vi "final_control_mk5_022625.vi"() -> ()   [LabVIEW 2023]
doc: "Simplified example program for initializing the COM port, determining the data frame of up to 26 Alicats, acquiring the data of the same number of Alicats, displaying the data of the one with the selected unit ID, and writing a setpoint to the same selected unit ID.\n\nThis is a slightly more feature rich version of the Alicat Simplified Driver Example, and contains an example of a method for interfacing with up to 26 Alicats on a single COM port by means of for loops with shift registers to handle sequential commands to each included Alicat. This also contains a method to write a setpoint to the same selected unit.\n\nIf coding for multiple Alicats on a single COM port without the use of for loops with shift registers, ensure that each Alicat command is executed sequentially. Alicat's RS-232/485 does not work if multiple devices are responding simultaneously."
uses:
  <vilib>/Platform/TimedLoop/XDataNode/timing_clust.ctl
  <vilib>/Platform/TimedLoop/XDataNode/nitl_modes.ctl
  <vilib>/Platform/TimedLoop/XDataNode/wakeup.ctl
  <vilib>/DAQmx/write.llb/DAQmx Write (Analog 1D DBL NChan 1Samp).vi
  <vilib>/DAQmx/read.llb/DAQmx Read (Analog 1D DBL 1Chan NSamp).vi
  <extravilib>/ChannelInstances/Tag-bool/Read With Abort.vi
  <extravilib>/ChannelInstances/Tag-bool/Write With Abort.vi
  <vilib>/Utility/file.llb/Write Delimited Spreadsheet (string).vi
  <extravilib>/ChannelInstances/Tag-bool/Instantiate.vi
  <vilib>/Utility/file.llb/Read Delimited Spreadsheet (DBL).vi
  <extravilib>/ChannelInstances/Tag-bool/EndpointRead.vi
  <vilib>/DAQmx/miscellaneous.llb/DAQmx Fill In Error Info.vi
  <extravilib>/ChannelInstances/Tag-bool/Endpoint.vi
  <vilib>/platform/TimedLoop/XDataNode/XDataNode.xnode
  <vilib>/Platform/TimedLoop/XDataNode/XDNodeRunTimeDep.lvlib
  <extravilib>/ChannelInstances/Tag-bool.lvlib
panel:
  in  "Tab Control":enum32{"Page 1", "Page 2"}(tab)
  in  "COM Port Settings":T1={"Baud Rate"=enum."19200", "VISA Sesssion In"="COM1"}
  out "Range Exceeded":bool
  out "Error Present":bool
  out "Error Text":string
  out "Elapsed Time [ms]\n(all units)":dbl caption="Elapsed Time (s)"
  in  "Minimum time between \nreadings [ms] (all units)":u32
  in  "Device ID's \nto Include:":T2={"A"=TRUE, "B"=TRUE, "C"=TRUE, "D"=TRUE, "E"=TRUE, "F"=TRUE, "G"=FALSE, "H"=FALSE, "I"=FALSE, "J"=FALSE, "K"=FALSE, "L"=FALSE, "M"=FALSE, "N"=FALSE, "O"=FALSE, "P"=FALSE, "Q"=FALSE, "R"=FALSE, "S"=FALSE, "T"=FALSE, "U"=FALSE, "V"=FALSE, "W"=FALSE, "X"=FALSE, "Y"=FALSE, "Z"=FALSE}
  out "Active Device":u16(ring) items=["A", "B", "C", "D", "E", "F"]
  out "Meas. Data (for active device)":T3
  in  "Write File":path=path "C:/Users/gtmiller/Downloads/Alicat LabVIEW 2014_2v1/Test.csv"
  in  "Hold Time [min]":dbl=17.0 min=17.0
  out "Global Start Time":i64
  out "N":i32
  out "Iteration Duration":i64
  in  "Read File":path
  in  "End Program":bool
  out "len_SP":i32
  out "Setpoints":dbl[][](array[numeric])=[[4.2, 3.3], [69.0, 4.2]]
  out "Z":dbl[](array[numeric])
  out "ASP":dbl
  out "BSP":dbl
  out "CSP":dbl
  out "DSP":dbl
  out "ESP":dbl
  out "FSP":dbl
  out "N_i_read":dbl
  out "N_read":i32
  out "read count":dbl=2.0
  out "T_SCh":string[](array[string])
  out "Iter_#":string
  out "V_D":string
  out "V_H":string
  out "Iter_Duration":string
  # "Totalizer Timer"
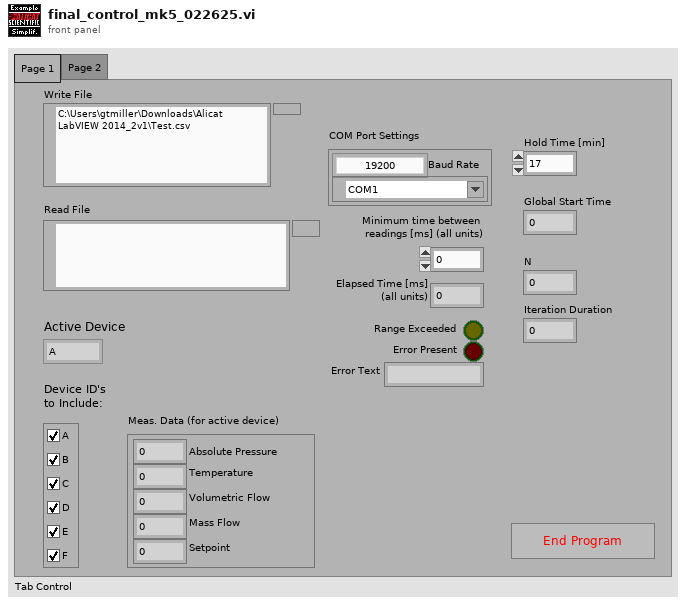
[diagram p1: front panel]
types:
  T1 = cluster{"Baud Rate":enum8{"2400", "9600", "19200", "38400", "57600", "115200", "Unknown"}, "VISA Sesssion In":refnum<visa-resource-name>}
  T2 = cluster{"A":bool, "B":bool, "C":bool, "D":bool, "E":bool, "F":bool, "G":bool, "H":bool, "I":bool, "J":bool, "K":bool, "L":bool, "M":bool, "N":bool, "O":bool, "P":bool, "Q":bool, "R":bool, "S":bool, "T":bool, "U":bool, "V":bool, "W":bool, "X":bool, "Y":bool, "Z":bool}
  T3 = cluster{"Absolute Pressure":dbl, "Gauge/Diff. Pressure":dbl, "Barometric Pressure":dbl, "Temperature":dbl, "Volumetric Flow":dbl, "Mass Flow":dbl, "Setpoint":dbl, "Valve Drive":dbl, "Totalizer":dbl, "[hr]":dbl, "[min]":dbl, "[sec]":dbl, "Totalizer Average Flow":dbl, "Totalizer Peak Flow":dbl, "Gas selected":string}
  T4 = cluster{"Unit ID":string, "Baud Rate":enum8{"2400", "9600", "19200", "38400", "57600", "115200", "Unknown"}, "VISA Sesssion In":refnum<visa-resource-name>}
  T5 = typedef "XDNodeRunTimeDep.lvlib/timing_clust.ctl" = cluster{"Expected End [f-1]":u64, "Actual End [f-1]":u64, "Finished Late? [f-1]":bool, "Expected End [i-1]":u64, "Actual End [i-1]":u64, "Finished Late? [i-1]":bool, "Expected Start [i]":u64, "Actual Start [i]":u64, "Expected Start [f]":u64, "Actual Start [f]":u64, "Source Name":string, "Structure Name":string, "Period":i64, "Deadline":i64, "Offset":i64, "Start":i64, "Priority":i32, "Timeout":i32, "Mode":T6, "Wakeup Reason":T7, "Error":errorcluster, "Source Type":string, "Secondary Source Type":string, "Global End Time":u64, "Global Start Time":u64, "Frame Duration":u64, "Iteration Duration":u64, "Assigned CPU":i32, "I/O Scan Engine Mode":u32}
  T6 = typedef "XDNodeRunTimeDep.lvlib/nitl_modes.ctl" = enum32{"No Change", "Process missed periods, maintain original phase", "Discard missed periods, maintain original phase", "Process missed periods, ignore original phase", "Discard missed periods, ignore original phase"}
  T7 = typedef "XDNodeRunTimeDep.lvlib/wakeup.ctl" = enum32{"Normal", "Aborted", "Asynchronous wakeup", "Timing source error", "Timed loop error", "Timeout"}
  T8 = typedef "Tag-bool.lvlib/))Channel.ctl" = refnum<queue>
  T9 = enum8{"2400", "9600", "19200", "38400", "57600", "115200", "Unknown"}
  T10 = cluster{"Absolute Pressure":bool, "Gauge/Diff. Pressure":bool, "Barometric Pressure":bool, "Temperature":bool, "Volumetric":bool, "Mass":bool, "Setpoint":bool, "Valve Drive":bool, "Totalizer":bool, "Totalizer Timer":bool, "Totalizer Average Flow":bool, "Totalizer Peak Flow":bool, "Gas Selected":bool, "Tot. Timer Format":u16}
  T11 = cluster{"Controller Full Scale":dbl, "Controller Select":u16, "Control Range":enum16{"Normal", "Inverted", "Bidirectional", "Unknown"}}
  T12 = cluster{"Controller Full Scale":dbl, "Controller Select":u16, "Control Range":enum16{"Normal", "Inverted", "Bidirectional", "Unknown"}}[]
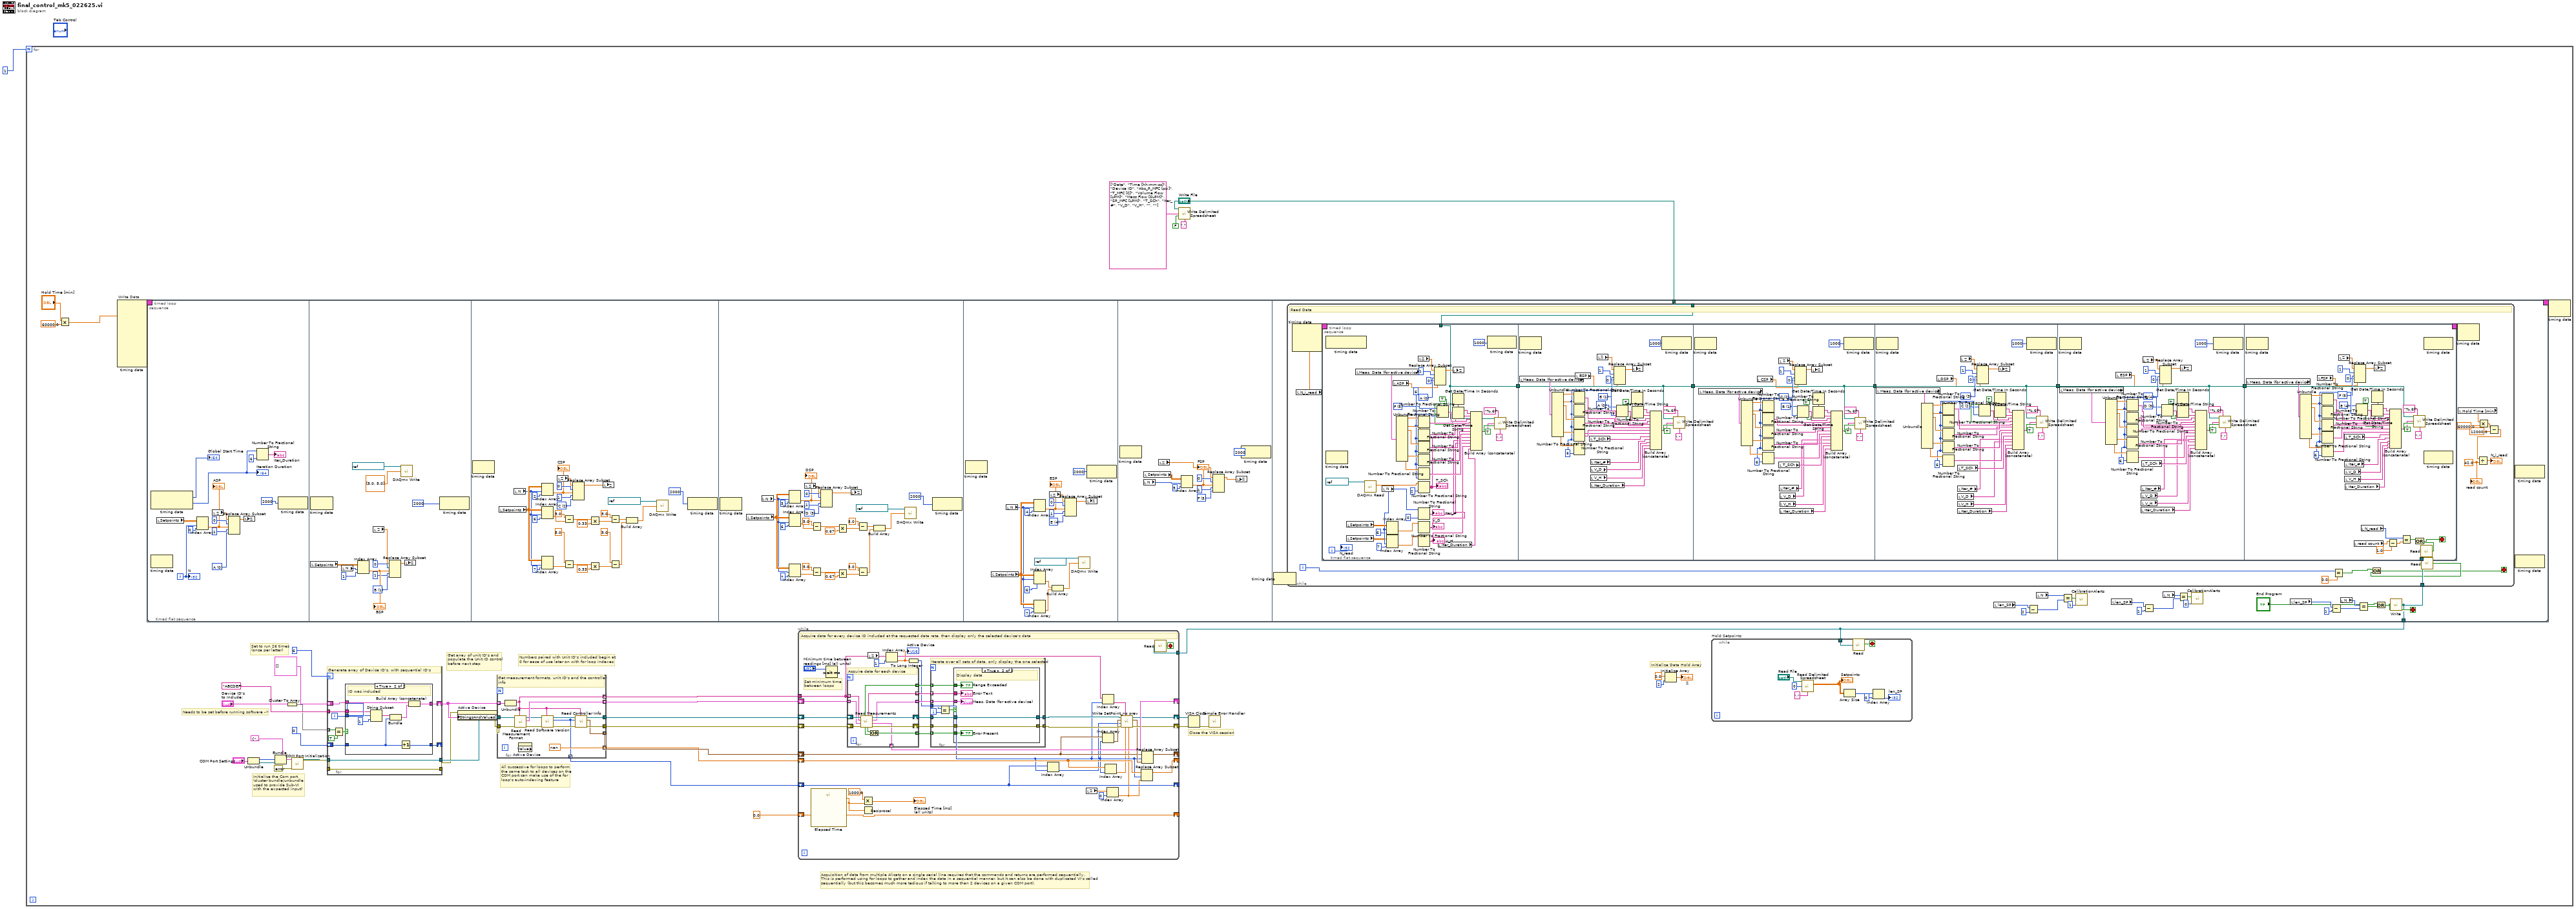
[diagram p0: block diagram]
diagram:
  n1 = for {
    N: 1 -> [_]
    # "Initialize Data Hold Array"
    # "All successive for loops to perform\nthe same task to all devices on the\nCOM port can make use of the for\nloop's auto-indexing feature"
    # "Set to run 26 times\n(once per letter)"
    # "Acquisition of data from multiple Alicats on a single serial line requires that the commands and returns are performed sequentially.\nThis is performed using for loops to gather and index the data in a sequential manner, but it can also be done with duplicated VI's called\nsequentially (but this becomes much more tedious if talking to more than 2 devices on a given COM port)."
    # "Numbers paired with Unit ID's included begin at\n0 for ease of use later on with for loop indexes"
    # "Get array of unit ID's and populate the Unit ID control before next step"
    # "Needs to be set before running software ->"
    # "Close the VISA session"
    # "Initialize the Com port\n(cluster bundle/unbundle\nused to provide Sub-VI \nwith the expected input)"
    n2 = Multiply(x="Hold Time [min]", y=60000.0) -> (x*y=w2:dbl)
    n3 = node-c288(w2) -> (w43:T5)  [unwired: 9 in]
    n4 = timed-loop "Write Data" {
      timing: w43 -> [_]
      timing-out: [_] -> w42
      tunnel: [w54] -> w9
      tunnel: "Write File" -> [w53]
      i -> [w68]
      stop <- w208 stop-if-true
      n5 = timed-sequence {
        timing: _ -> [_]
        timing-out: _ -> [_]
        tunnel: [w56] -> w54
        tunnel: w53 -> [w55]
        n6 = timed-flat-sequence {
          tunnel: [w203] -> w56
          tunnel: w55 -> [w204]
          frame #0 {
            w61 = u16 0 items=["A", "B", "C", "D", "E", "F"]
            n7 = node-c288() -> (→"Global Start Time":i64, w60:i64)  [unwired: 1 in]
            "Iteration Duration" <- w60
            n8 = local read "Setpoints"() -> (w70:dbl[][])
            n9 = Index Array(array=w70, index (row)=w68, index (col)=0 ("index (row)")) -> (element=w66:dbl)
            "ASP" <- w66
            n10 = local read "Z"() -> (w64:dbl[])
            n11 = Replace Array Subset(array=w64, new element #1=w66, index #1=0 ("index"), new element #2=w61, index #2=1 ("index")) -> (w65:dbl[])
            n12 = local write "Z"(w65) -> ()
            n13 = Number To Fractional String(number=w60, precision (6)=i16 6) -> (F-format string=→"Iter_Duration":string)  [unwired: 2 in]
            n14 = node-c288(i64 2000 ("Start")) -> ()  [unwired: 1 out]
            "N" <- w68
          }
          frame #1 {
            w79 = u16 1 items=["A", "B", "C", "D", "E", "F"]
            n15 = node-c288() -> ()  [unwired: 1 in, 1 out]
            n16 = local read "Setpoints"() -> (w87:dbl[][])
            n17 = local read "N"() -> (w80:i32)
            n18 = Index Array(array=w87, index (row)=w80, index (col)=1 ("index (row)")) -> (element=w84:dbl)
            "BSP" <- w84
            n19 = local read "Z"() -> (w82:dbl[])
            n20 = Replace Array Subset(array=w82, new element #1=w84, index #1=0 ("index"), new element #2=w79, index #2=1 ("index")) -> (w83:dbl[])
            n21 = call-poly <vilib>:"DAQmx Write.vi"("task/channels in"=refnum<k21> "Valve_cont", "data"=dbl[] [5.0, 5.0]) -> ()  [unwired: 11 in, 3 out]
            n22 = local write "Z"(w83) -> ()
            n23 = node-c288(i64 2000 ("Start")) -> ()  [unwired: 1 out]
          }
          frame #2 {
            w113 = u16 2 items=["A", "B", "C", "D", "E", "F"]
            n24 = node-c288() -> ()  [unwired: 1 in, 1 out]
            n25 = local read "Setpoints"() -> (w96:dbl[][])
            n26 = local read "N"() -> (w95:i32)
            n27 = Index Array(array=w96, index (row)=w95, index (col)=2 ("index (row)")) -> (element=w117:dbl)
            "CSP" <- w117
            n28 = Index Array(array=w96, index (row)=w95, index (col)=6 ("disabled index (col)")) -> (element=w94:dbl)
            n29 = Index Array(array=w96, index (row)=w95, index (col)=7 ("disabled index (col)")) -> (element=w93:dbl)
            n30 = local read "Z"() -> (w115:dbl[])
            n31 = Subtract(x=5.0, y=w94) -> (x-y=w110:dbl)
            n32 = Subtract(x=5.0, y=w93) -> (x-y=w105:dbl)
            n33 = Replace Array Subset(array=w115, new element #1=w117, index #1=0 ("index"), new element #2=w113, index #2=1 ("index")) -> (w116:dbl[])
            n34 = Multiply(x=w110, y=0.33) -> (x*y=w108:dbl)
            n35 = Multiply(x=w105, y=0.33) -> (x*y=w103:dbl)
            n36 = local write "Z"(w116) -> ()
            n37 = Subtract(x=5.0, y=w108) -> (x-y=w98:dbl)
            n38 = Subtract(x=5.0, y=w103) -> (x-y=w99:dbl)
            n39 = Build Array(w98, w99) -> (w97:dbl[])
            n40 = call-poly <vilib>:"DAQmx Write.vi"("task/channels in"=refnum<k21> "Valve_cont", "data"=w97) -> ()  [unwired: 11 in, 3 out]
            n41 = node-c288(i64 2000 ("Start")) -> ()  [unwired: 1 out]
          }
          frame #3 {
            w145 = u16 3 items=["A", "B", "C", "D", "E", "F"]
            n42 = node-c288() -> ()  [unwired: 1 in, 1 out]
            n43 = local read "Setpoints"() -> (w128:dbl[][])
            n44 = local read "N"() -> (w127:i32)
            n45 = Index Array(array=w128, index (row)=w127, index (col)=3 ("index (row)")) -> (element=w149:dbl)
            "DSP" <- w149
            n46 = Index Array(array=w128, index (row)=w127, index (col)=6 ("disabled index (col)")) -> (element=w126:dbl)
            n47 = Index Array(array=w128, index (row)=w127, index (col)=7 ("disabled index (col)")) -> (element=w125:dbl)
            n48 = local read "Z"() -> (w147:dbl[])
            n49 = Subtract(x=5.0, y=w126) -> (x-y=w142:dbl)
            n50 = Subtract(x=5.0, y=w125) -> (x-y=w137:dbl)
            n51 = Replace Array Subset(array=w147, new element #1=w149, index #1=0 ("index"), new element #2=w145, index #2=1 ("index")) -> (w148:dbl[])
            n52 = Multiply(x=w142, y=0.67) -> (x*y=w140:dbl)
            n53 = Multiply(x=w137, y=0.67) -> (x*y=w135:dbl)
            n54 = local write "Z"(w148) -> ()
            n55 = Subtract(x=5.0, y=w140) -> (x-y=w130:dbl)
            n56 = Subtract(x=5.0, y=w135) -> (x-y=w131:dbl)
            n57 = Build Array(w130, w131) -> (w129:dbl[])
            n58 = call-poly <vilib>:"DAQmx Write.vi"("task/channels in"=refnum<k21> "Valve_cont", "data"=w129) -> ()  [unwired: 11 in, 3 out]
            n59 = node-c288(i64 2000 ("Start")) -> ()  [unwired: 1 out]
          }
          frame #4 {
            w166 = u16 4 items=["A", "B", "C", "D", "E", "F"]
            n60 = node-c288() -> ()  [unwired: 1 in, 1 out]
            n61 = local read "Setpoints"() -> (w160:dbl[][])
            n62 = local read "N"() -> (w159:i32)
            n63 = Index Array(array=w160, index (row)=w159, index (col)=4 ("index (row)")) -> (element=w170:dbl)
            "ESP" <- w170
            n64 = Index Array(array=w160, index (row)=w159, index (col)=6 ("disabled index (col)")) -> (element=w162:dbl)
            n65 = Index Array(array=w160, index (row)=w159, index (col)=7 ("disabled index (col)")) -> (element=w161:dbl)
            n66 = local read "Z"() -> (w168:dbl[])
            n67 = Build Array(w162, w161) -> (w158:dbl[])
            n68 = Replace Array Subset(array=w168, new element #1=w170, index #1=0 ("index"), new element #2=w166, index #2=1 ("index")) -> (w169:dbl[])
            n69 = call-poly <vilib>:"DAQmx Write.vi"("task/channels in"=refnum<k21> "Valve_cont", "data"=w158) -> ()  [unwired: 11 in, 3 out]
            n70 = local write "Z"(w169) -> ()
            n71 = node-c288(i64 2000 ("Start")) -> ()  [unwired: 1 out]
          }
          frame #5 {
            w180 = u16 5 items=["A", "B", "C", "D", "E", "F"]
            n72 = node-c288() -> ()  [unwired: 1 in, 1 out]
            n73 = local read "N"() -> (w178:i32)
            n74 = local read "Setpoints"() -> (w183:dbl[][])
            n75 = local read "Z"() -> (w182:dbl[])
            n76 = Index Array(array=w183, index (row)=w178, index (col)=5 ("index (row)")) -> (element=w179:dbl)
            "FSP" <- w179
            n77 = Replace Array Subset(array=w182, new element #1=w179, index #1=0 ("index"), new element #2=w180, index #2=1 ("index")) -> (w181:dbl[])
            n78 = local write "Z"(w181) -> ()
            n79 = node-c288(i64 2000 ("Start")) -> ()  [unwired: 1 out]
          }
          frame #6 {
            n80 = node-c288() -> ()  [unwired: 1 in, 1 out]
            n81 = local read "len_SP"() -> (w192:i32)
            n82 = Subtract(x=w192, y=2) -> (x-y=w194:i32)
            n83 = local read "N"() -> (w193:i32)
            n84 = Equal?(x=w193, y=w194) -> (x = y?=w195:bool)
            n85 = call "CalibrationAlerts.vi"("Alert Type (0)"=1, "Trigger"=w195) -> ()  [unwired: 10 in]
            n86 = local read "len_SP"() -> (w198:i32)
            n87 = Subtract(x=w198, y=1) -> (x-y=w197:i32)
            n88 = local read "N"() -> (w202:i32)
            n89 = Equal?(x=w202, y=w197) -> (x = y?=w200:bool)
            n90 = call "CalibrationAlerts.vi"("Alert Type (0)"=0, "Trigger"=w200) -> ()  [unwired: 10 in]
            n91 = local read "len_SP"() -> (w207:i32)
            n92 = Subtract(x=w207, y=1) -> (x-y=w210:i32)
            n93 = local read "N"() -> (w206:i32)
            n94 = Equal?(x=w206, y=w210) -> (x = y?=w209:bool)
            n95 = Or(x="End Program", y=w209) -> (x .or. y?=w208:bool)
            n96 = call <extravilib>:"Write.vi"("element"=w208) -> ("channel"=w203:T8)  [unwired: 1 out]
            n97 = while {
              tunnel: w204 -> [w226]
              tunnel: w203 -> [w220]
              i -> [w216]
              stop <- w215 stop-if-true
              w221 = 42.0 ("y")
              # "Read Data"
              n98 = local read "N_i_read"() -> (w213:dbl)
              n99 = node-c288(w213) -> (w228:T5)  [unwired: 2 in]
              n100 = timed-loop {
                timing: w228 -> [_]
                timing-out: [_] -> w227
                tunnel: w226 -> [w230]
                tunnel: w220 -> [w229]
                i -> [w256]
                stop <- w455 stop-if-true
                n101 = timed-sequence {
                  timing: _ -> [_]
                  timing-out: _ -> [_]
                  tunnel: w230 -> [w237]
                  tunnel: w229 -> [w231]
                  n102 = timed-flat-sequence {
                    tunnel: w237 -> [w259]
                    tunnel: [w259] -> w236
                    tunnel: w236 -> [w298]
                    tunnel: [w298] -> w235
                    tunnel: w235 -> [w337]
                    tunnel: [w337] -> w234
                    tunnel: w234 -> [w376]
                    tunnel: [w376] -> w233
                    tunnel: w233 -> [w415]
                    tunnel: [w415] -> w232
                    tunnel: w232 -> [w462]
                    tunnel: w231 -> [w461]
                    frame #0 {
                      w255 = u16 5 items=["A", "B", "C", "D", "E", "F"]
                      w262 = u16 0 items=["A", "B", "C", "D", "E", "F"]
                      w263 = i16 6 ("precision (6)")
                      n103 = node-c288() -> ()  [unwired: 1 in, 1 out]
                      n104 = local read "Setpoints"() -> (w249:dbl[][])
                      n105 = local read "Setpoints"() -> (w245:dbl[][])
                      n106 = local read "Meas. Data (for active device)"() -> (w270:T3)
                      n107 = call-poly <vilib>:"DAQmx Read.vi"("task/channels in"=refnum<k21> "T_SCh") -> ("data"=w253:dbl[])  [unwired: 12 in, 2 out]
                      n108 = local read "N"() -> (w246:i32)
                      n109 = Index Array(array=w249, index (row)=w246, index (col)=6 ("disabled index (col)")) -> (element=w248:dbl)
                      n110 = Index Array(array=w245, index (row)=w246, index (col)=7 ("disabled index (col)")) -> (element=w247:dbl)
                      n111 = local read "ASP"() -> (w257:dbl)
                      n112 = Unbundle(w270) -> ("Absolute Pressure"=w283:dbl, "Temperature"=w279:dbl, "Volumetric Flow"=w269:dbl, "Mass Flow"=w280:dbl, "Setpoint"=w281:dbl)  [unwired: 10 out]
                      n113 = local read "Z"() -> (w266:dbl[])
                      n114 = Number To Fractional String(number=w283, precision (6)=w263) -> (F-format string=w278:string)  [unwired: 2 in]
                      n115 = Number To Fractional String(number=w279, precision (6)=w263) -> (F-format string=w277:string)  [unwired: 2 in]
                      n116 = Number To Fractional String(number=w269, precision (6)=w263) -> (F-format string=w276:string)  [unwired: 2 in]
                      n117 = Number To Fractional String(number=w280, precision (6)=w263) -> (F-format string=w275:string)  [unwired: 2 in]
                      n118 = Number To Fractional String(number=w281, precision (6)=w263) -> (F-format string=w274:string)  [unwired: 2 in]
                      n119 = Number To Fractional String(number=w253, precision (6)=i16 2) -> (F-format string=w252:string[])  [unwired: 2 in]
                      "T_SCh" <- w252
                      n120 = Number To Fractional String(number=w246, precision (6)=i16 0) -> (F-format string=w241:string)  [unwired: 2 in]
                      "Iter_#" <- w241
                      n121 = Number To Fractional String(number=w248) -> (F-format string=w240:string)  [unwired: 3 in]
                      "V_D" <- w240
                      n122 = Number To Fractional String(number=w247) -> (F-format string=w239:string)  [unwired: 3 in]
                      "V_H" <- w239
                      n123 = Replace Array Subset(array=w266, new element #1=w262, index #1=1 ("index"), new element #2=w257, index #2=0 ("index")) -> (w264:dbl[])
                      n124 = Number To Fractional String(number=w255, precision (6)=w263) -> (F-format string=w282:string)  [unwired: 2 in]
                      n125 = local read "Iter_Duration"() -> (w238:string)
                      n126 = Get Date/Time In Seconds() -> (seconds since 1Jan1904=w268:timestamp)
                      n127 = Get Date/Time String(seconds (now)=w268, want seconds? (F)=TRUE) -> (date string=w267:string, time string=w284:string)  [unwired: 1 in]
                      n128 = local write "Z"(w264) -> ()
                      n129 = Build Array (concatenate)(w267, w284, w282, w278, w277, w276, w275, w274, w252, w241, w240, w239, w238) -> (w271:string[])
                      n130 = node-c288(i64 1000 ("Start")) -> ()  [unwired: 1 out]
                      n131 = call-poly <vilib>:"Write Delimited Spreadsheet.vi"("file path (dialog if empty)"=w259, "format (%s)"="%.6f" ("format (%.3f)"), "1D data"=w271, "append to file? (new file:F)"=TRUE, "delimiter (\\t)"="," ("delimiter (\\t)")) -> ()  [unwired: 9 in, 2 out]
                      "N_read" <- w256
                    }
                    frame #1 {
                      w295 = u16 0 items=["A", "B", "C", "D", "E", "F"]
                      w304 = u16 1 items=["A", "B", "C", "D", "E", "F"]
                      w305 = i16 6 ("precision (6)")
                      n132 = node-c288() -> ()  [unwired: 1 in, 1 out]
                      n133 = local read "Meas. Data (for active device)"() -> (w302:T3)
                      n134 = Unbundle(w302) -> ("Absolute Pressure"=w322:dbl, "Temperature"=w318:dbl, "Volumetric Flow"=w309:dbl, "Mass Flow"=w319:dbl, "Setpoint"=w320:dbl)  [unwired: 10 out]
                      n135 = Number To Fractional String(number=w322, precision (6)=w305) -> (F-format string=w317:string)  [unwired: 2 in]
                      n136 = Number To Fractional String(number=w318, precision (6)=w305) -> (F-format string=w316:string)  [unwired: 2 in]
                      n137 = Number To Fractional String(number=w309, precision (6)=w305) -> (F-format string=w315:string)  [unwired: 2 in]
                      n138 = Number To Fractional String(number=w319, precision (6)=w305) -> (F-format string=w314:string)  [unwired: 2 in]
                      n139 = Number To Fractional String(number=w320, precision (6)=w305) -> (F-format string=w313:string)  [unwired: 2 in]
                      n140 = local read "BSP"() -> (w296:dbl)
                      n141 = local read "T_SCh"() -> (w294:string[])
                      n142 = local read "Iter_#"() -> (w292:string)
                      n143 = local read "V_D"() -> (w291:string)
                      n144 = local read "V_H"() -> (w290:string)
                      n145 = local read "Iter_Duration"() -> (w289:string)
                      n146 = local read "Z"() -> (w301:dbl[])
                      n147 = Replace Array Subset(array=w301, new element #1=w304, index #1=1 ("index"), new element #2=w296, index #2=0 ("index")) -> (w300:dbl[])
                      n148 = Number To Fractional String(number=w295, precision (6)=w305) -> (F-format string=w321:string)  [unwired: 2 in]
                      n149 = Get Date/Time In Seconds() -> (seconds since 1Jan1904=w308:timestamp)
                      n150 = Get Date/Time String(seconds (now)=w308, want seconds? (F)=TRUE) -> (date string=w307:string, time string=w323:string)  [unwired: 1 in]
                      n151 = local write "Z"(w300) -> ()
                      n152 = Build Array (concatenate)(w307, w323, w321, w317, w316, w315, w314, w313, w294, w292, w291, w290, w289) -> (w310:string[])
                      n153 = node-c288(i64 1000 ("Start")) -> ()  [unwired: 1 out]
                      n154 = call-poly <vilib>:"Write Delimited Spreadsheet.vi"("file path (dialog if empty)"=w298, "format (%s)"="%.6f" ("format (%.3f)"), "1D data"=w310, "append to file? (new file:F)"=TRUE, "delimiter (\\t)"="," ("delimiter (\\t)")) -> ()  [unwired: 9 in, 2 out]
                    }
                    frame #2 {
                      w334 = u16 1 items=["A", "B", "C", "D", "E", "F"]
                      w343 = u16 2 items=["A", "B", "C", "D", "E", "F"]
                      w344 = i16 6 ("precision (6)")
                      n155 = node-c288() -> ()  [unwired: 1 in, 1 out]
                      n156 = local read "Meas. Data (for active device)"() -> (w339:T3)
                      n157 = Unbundle(w339) -> ("Absolute Pressure"=w361:dbl, "Temperature"=w357:dbl, "Volumetric Flow"=w348:dbl, "Mass Flow"=w358:dbl, "Setpoint"=w359:dbl)  [unwired: 10 out]
                      n158 = local read "CSP"() -> (w335:dbl)
                      n159 = Number To Fractional String(number=w361, precision (6)=w344) -> (F-format string=w356:string)  [unwired: 2 in]
                      n160 = Number To Fractional String(number=w357, precision (6)=w344) -> (F-format string=w355:string)  [unwired: 2 in]
                      n161 = Number To Fractional String(number=w348, precision (6)=w344) -> (F-format string=w354:string)  [unwired: 2 in]
                      n162 = Number To Fractional String(number=w358, precision (6)=w344) -> (F-format string=w353:string)  [unwired: 2 in]
                      n163 = Number To Fractional String(number=w359, precision (6)=w344) -> (F-format string=w352:string)  [unwired: 2 in]
                      n164 = local read "Z"() -> (w341:dbl[])
                      n165 = local read "T_SCh"() -> (w333:string[])
                      n166 = local read "Iter_#"() -> (w331:string)
                      n167 = local read "V_D"() -> (w330:string)
                      n168 = local read "V_H"() -> (w329:string)
                      n169 = local read "Iter_Duration"() -> (w328:string)
                      n170 = Replace Array Subset(array=w341, new element #1=w343, index #1=1 ("index"), new element #2=w335, index #2=0 ("index")) -> (w340:dbl[])
                      n171 = Number To Fractional String(number=w334, precision (6)=w344) -> (F-format string=w360:string)  [unwired: 2 in]
                      n172 = local write "Z"(w340) -> ()
                      n173 = Get Date/Time In Seconds() -> (seconds since 1Jan1904=w347:timestamp)
                      n174 = Get Date/Time String(seconds (now)=w347, want seconds? (F)=TRUE) -> (date string=w346:string, time string=w362:string)  [unwired: 1 in]
                      n175 = Build Array (concatenate)(w346, w362, w360, w356, w355, w354, w353, w352, w333, w331, w330, w329, w328) -> (w349:string[])
                      n176 = node-c288(i64 1000 ("Start")) -> ()  [unwired: 1 out]
                      n177 = call-poly <vilib>:"Write Delimited Spreadsheet.vi"("file path (dialog if empty)"=w337, "format (%s)"="%.6f" ("format (%.3f)"), "1D data"=w349, "append to file? (new file:F)"=TRUE, "delimiter (\\t)"="," ("delimiter (\\t)")) -> ()  [unwired: 9 in, 2 out]
                    }
                    frame #3 {
                      w373 = u16 2 items=["A", "B", "C", "D", "E", "F"]
                      w382 = u16 3 items=["A", "B", "C", "D", "E", "F"]
                      w383 = i16 6 ("precision (6)")
                      n178 = node-c288() -> ()  [unwired: 1 in, 1 out]
                      n179 = local read "Meas. Data (for active device)"() -> (w380:T3)
                      n180 = Unbundle(w380) -> ("Absolute Pressure"=w400:dbl, "Temperature"=w396:dbl, "Volumetric Flow"=w387:dbl, "Mass Flow"=w397:dbl, "Setpoint"=w398:dbl)  [unwired: 10 out]
                      n181 = local read "DSP"() -> (w374:dbl)
                      n182 = Number To Fractional String(number=w400, precision (6)=w383) -> (F-format string=w395:string)  [unwired: 2 in]
                      n183 = Number To Fractional String(number=w396, precision (6)=w383) -> (F-format string=w394:string)  [unwired: 2 in]
                      n184 = Number To Fractional String(number=w387, precision (6)=w383) -> (F-format string=w393:string)  [unwired: 2 in]
                      n185 = Number To Fractional String(number=w397, precision (6)=w383) -> (F-format string=w392:string)  [unwired: 2 in]
                      n186 = Number To Fractional String(number=w398, precision (6)=w383) -> (F-format string=w391:string)  [unwired: 2 in]
                      n187 = local read "T_SCh"() -> (w372:string[])
                      n188 = local read "Iter_#"() -> (w370:string)
                      n189 = local read "V_D"() -> (w369:string)
                      n190 = local read "V_H"() -> (w368:string)
                      n191 = local read "Iter_Duration"() -> (w367:string)
                      n192 = local read "Z"() -> (w379:dbl[])
                      n193 = Replace Array Subset(array=w379, new element #1=w382, index #1=1 ("index"), new element #2=w374, index #2=0 ("index")) -> (w378:dbl[])
                      n194 = Number To Fractional String(number=w373, precision (6)=w383) -> (F-format string=w399:string)  [unwired: 2 in]
                      n195 = Get Date/Time In Seconds() -> (seconds since 1Jan1904=w386:timestamp)
                      n196 = Get Date/Time String(seconds (now)=w386, want seconds? (F)=TRUE) -> (date string=w385:string, time string=w401:string)  [unwired: 1 in]
                      n197 = local write "Z"(w378) -> ()
                      n198 = Build Array (concatenate)(w385, w401, w399, w395, w394, w393, w392, w391, w372, w370, w369, w368, w367) -> (w388:string[])
                      n199 = node-c288(i64 1000 ("Start")) -> ()  [unwired: 1 out]
                      n200 = call-poly <vilib>:"Write Delimited Spreadsheet.vi"("file path (dialog if empty)"=w376, "format (%s)"="%.6f" ("format (%.3f)"), "1D data"=w388, "append to file? (new file:F)"=TRUE, "delimiter (\\t)"="," ("delimiter (\\t)")) -> ()  [unwired: 9 in, 2 out]
                    }
                    frame #4 {
                      w412 = u16 3 items=["A", "B", "C", "D", "E", "F"]
                      w421 = u16 4 items=["A", "B", "C", "D", "E", "F"]
                      w422 = i16 6 ("precision (6)")
                      n201 = node-c288() -> ()  [unwired: 1 in, 1 out]
                      n202 = local read "Meas. Data (for active device)"() -> (w419:T3)
                      n203 = Unbundle(w419) -> ("Absolute Pressure"=w439:dbl, "Temperature"=w435:dbl, "Volumetric Flow"=w426:dbl, "Mass Flow"=w436:dbl, "Setpoint"=w437:dbl)  [unwired: 10 out]
                      n204 = local read "ESP"() -> (w413:dbl)
                      n205 = Number To Fractional String(number=w439, precision (6)=w422) -> (F-format string=w434:string)  [unwired: 2 in]
                      n206 = Number To Fractional String(number=w435, precision (6)=w422) -> (F-format string=w433:string)  [unwired: 2 in]
                      n207 = Number To Fractional String(number=w426, precision (6)=w422) -> (F-format string=w432:string)  [unwired: 2 in]
                      n208 = Number To Fractional String(number=w436, precision (6)=w422) -> (F-format string=w431:string)  [unwired: 2 in]
                      n209 = Number To Fractional String(number=w437, precision (6)=w422) -> (F-format string=w430:string)  [unwired: 2 in]
                      n210 = local read "Iter_Duration"() -> (w406:string)
                      n211 = local read "Iter_#"() -> (w409:string)
                      n212 = local read "V_D"() -> (w408:string)
                      n213 = local read "V_H"() -> (w407:string)
                      n214 = local read "T_SCh"() -> (w411:string[])
                      n215 = local read "Z"() -> (w418:dbl[])
                      n216 = Replace Array Subset(array=w418, new element #1=w421, index #1=1 ("index"), new element #2=w413, index #2=0 ("index")) -> (w417:dbl[])
                      n217 = Number To Fractional String(number=w412, precision (6)=w422) -> (F-format string=w438:string)  [unwired: 2 in]
                      n218 = Get Date/Time In Seconds() -> (seconds since 1Jan1904=w425:timestamp)
                      n219 = Get Date/Time String(seconds (now)=w425, want seconds? (F)=TRUE) -> (date string=w424:string, time string=w440:string)  [unwired: 1 in]
                      n220 = local write "Z"(w417) -> ()
                      n221 = Build Array (concatenate)(w424, w440, w438, w434, w433, w432, w431, w430, w411, w409, w408, w407, w406) -> (w427:string[])
                      n222 = node-c288(i64 1000 ("Start")) -> ()  [unwired: 1 out]
                      n223 = call-poly <vilib>:"Write Delimited Spreadsheet.vi"("file path (dialog if empty)"=w415, "format (%s)"="%.6f" ("format (%.3f)"), "1D data"=w427, "append to file? (new file:F)"=TRUE, "delimiter (\\t)"="," ("delimiter (\\t)")) -> ()  [unwired: 9 in, 2 out]
                    }
                    frame #5 {
                      w451 = u16 4 items=["A", "B", "C", "D", "E", "F"]
                      w467 = u16 5 items=["A", "B", "C", "D", "E", "F"]
                      w468 = i16 6 ("precision (6)")
                      n224 = node-c288() -> ()  [unwired: 1 in, 1 out]
                      n225 = local read "Meas. Data (for active device)"() -> (w465:T3)
                      n226 = Unbundle(w465) -> ("Absolute Pressure"=w485:dbl, "Temperature"=w481:dbl, "Volumetric Flow"=w472:dbl, "Mass Flow"=w482:dbl, "Setpoint"=w483:dbl)  [unwired: 10 out]
                      n227 = local read "FSP"() -> (w459:dbl)
                      n228 = Number To Fractional String(number=w485, precision (6)=w468) -> (F-format string=w480:string)  [unwired: 2 in]
                      n229 = Number To Fractional String(number=w481, precision (6)=w468) -> (F-format string=w479:string)  [unwired: 2 in]
                      n230 = Number To Fractional String(number=w472, precision (6)=w468) -> (F-format string=w478:string)  [unwired: 2 in]
                      n231 = Number To Fractional String(number=w482, precision (6)=w468) -> (F-format string=w477:string)  [unwired: 2 in]
                      n232 = Number To Fractional String(number=w483, precision (6)=w468) -> (F-format string=w476:string)  [unwired: 2 in]
                      n233 = local read "Z"() -> (w464:dbl[])
                      n234 = local read "T_SCh"() -> (w450:string[])
                      n235 = local read "Iter_#"() -> (w448:string)
                      n236 = local read "V_D"() -> (w447:string)
                      n237 = local read "V_H"() -> (w446:string)
                      n238 = local read "Iter_Duration"() -> (w445:string)
                      n239 = Replace Array Subset(array=w464, new element #1=w467, index #1=1 ("index"), new element #2=w459, index #2=0 ("index")) -> (w463:dbl[])
                      n240 = local read "read count"() -> (w452:dbl)
                      n241 = Number To Fractional String(number=w451, precision (6)=w468) -> (F-format string=w484:string)  [unwired: 2 in]
                      n242 = local read "N_read"() -> (w456:i32)
                      n243 = Get Date/Time In Seconds() -> (seconds since 1Jan1904=w471:timestamp)
                      n244 = Get Date/Time String(seconds (now)=w471, want seconds? (F)=TRUE) -> (date string=w470:string, time string=w486:string)  [unwired: 1 in]
                      n245 = local write "Z"(w463) -> ()
                      n246 = Subtract(x=w452, y=1.0) -> (x-y=w454:dbl)
                      n247 = Build Array (concatenate)(w470, w486, w484, w480, w479, w478, w477, w476, w450, w448, w447, w446, w445) -> (w473:string[])
                      n248 = Equal?(x=w456, y=w454) -> (x = y?=w457:bool)
                      n249 = call-poly <vilib>:"Write Delimited Spreadsheet.vi"("file path (dialog if empty)"=w462, "format (%s)"="%.6f" ("format (%.3f)"), "1D data"=w473, "append to file? (new file:F)"=TRUE, "delimiter (\\t)"="," ("delimiter (\\t)")) -> ()  [unwired: 9 in, 2 out]
                      n250 = call <extravilib>:"Read.vi"("channel"=w461) -> ("element"=w458:bool)  [unwired: 1 in, 1 out]
                      n251 = Or(x=w457, y=w458) -> (x .or. y?=w455:bool)
                      n252 = node-c288() -> ()  [unwired: 1 in, 1 out]
                    }
                  }
                }
                n253 = node-c288() -> ()  [unwired: 1 in, 1 out]
                n254 = node-c288() -> ()  [unwired: 1 in, 1 out]
              }
              n255 = Equal?(x=w216, y=0.0) -> (x = y?=w218:bool)
              n256 = call <extravilib>:"Read.vi"("channel"=w220) -> ("element"=w217:bool)  [unwired: 1 in, 1 out]
              n257 = Or(x=w218, y=w217) -> (x .or. y?=w215:bool)
              n258 = node-c288(w227) -> ()  [unwired: 1 out]
              n259 = local read "Hold Time [min]"() -> (w224:dbl)
              n260 = Multiply(x=w224, y=60000.0) -> (x*y=w223:dbl)
              n261 = Subtract(x=w223, y=12000.0) -> (x-y=w214:dbl)
              n262 = Divide(x=w214, y=w221) -> (x/y=→"N_i_read":dbl)
              "read count" <- w221
            }
            n263 = node-c288() -> ()  [unwired: 1 in, 1 out]
          }
        }
      }
      n264 = node-c288() -> ()  [unwired: 1 in, 1 out]
      n265 = node-c288() -> ()  [unwired: 1 in, 1 out]
    }
    n266 = Unbundle("COM Port Settings") -> ("Baud Rate"=w34:T9, "VISA Sesssion In"=w33:refnum<visa-resource-name>)
    n267 = Bundle(cluster=T4 {"Unit ID"="A", "Baud Rate"=enum."19200", "VISA Sesssion In"="COM1"} ("Communication Settings"), "Baud Rate"=w34, "VISA Sesssion In"=w33) -> (w32:T4)  [unwired: 1 in]
    n268 = Cluster To Array(cluster="Device ID's \nto Include:") -> (array=w28:bool[])
    n269 = call "COM Port Initialization.vi"("error in (no error)"=errorcluster {"status"=FALSE, "code"=0, "source"=""}, "Communication Settings"=w32) -> ("error out"=w25:errorcluster, "VISA Session Out"=w24:refnum<visa-resource-name>)  [unwired: 8 in]
    n270 = for {
      N: 6 -> [_]
      tunnel: "ABCDEF" -> [w527]
      tunnel: w28 -> [w520] mode=indexing
      shift-right: [w519] -> _
      shift-left: u16 0 ("length (rest)") -> [w525]
      shift-right: [w524] -> w22
      shift-left: cluster{string, u16}[] [] -> [w523]
      tunnel: w25 -> [w518]
      tunnel: w24 -> [w517]
      tunnel: [w518] -> w15
      tunnel: [w517] -> w23
      i -> [w526]
      # "Generate array of Device ID's, with sequential ID's"
      n271 = Equal?(x=w520, y=TRUE) -> (x = y?=w522:bool)
      n272 = case shown="True" w522 {
        tunnel: w527 -> [_ w538]
        tunnel: w526 -> [_ w537]
        tunnel: w525 -> [w528 w530]
        tunnel: [w529 w533] -> w524
        tunnel: w523 -> [w529 w531]
        tunnel: [w528 w534] -> w519
        frame False {
          # "ID was not included"
        }
        frame True {
          # "ID was included"
          n273 = String Subset(string=w538, offset (0)=w537, length (rest)=1 ("length (rest)")) -> (substring=w535:string)
          n274 = Bundle(w535, "length (rest)"=w530) -> (w532:cluster{string, "length (rest)":u16})  [unwired: 1 in]
          n275 = Increment(x=w530) -> (x+1=w534:u16)
          n276 = Build Array (concatenate)(w531, w532) -> (w533:cluster{string, "length (rest)":u16}[])
        }
      }
    }
    n277 = property on="Active Device" class="Ring (strict)"(error in=w15, "StringsAndValues[]"=w22) -> (error out=w14:errorcluster)  [unwired: 1 in, 1 out]
    n278 = for {
      tunnel: w23 -> [w515]
      tunnel: [w512] -> w19
      tunnel: w14 -> [w516]
      tunnel: [w511] -> w18
      tunnel: w22 -> [w513] mode=indexing
      tunnel: [w514] -> w21 mode=indexing
      tunnel: [w504] -> w20 mode=indexing
      tunnel: [w510] -> w17 mode=indexing
      tunnel: [nan ("Setpoint")] -> w16 mode=indexing
      tunnel: [w503] -> w13 mode=indexing
      # "Get measurement formats, unit ID's and the controller info"
      n279 = Unbundle(w513) -> (w504:string)  [unwired: 1 out]
      n280 = call "Read Measurement Format.vi"("Unit ID (A)"=w504, "error in"=w516, "VISA Session In"=w515) -> ("error out"=w507:errorcluster, "Data Frame Format"=w514:T10, "VISA Session Out"=w508:refnum<visa-resource-name>)  [unwired: 6 in]
      n281 = property on="Active Device" class="Ring (strict)" props=["Value"]() -> ()  [unwired: 2 in, 3 out]
      n282 = call "Read Software Version.vi"("Unit ID (A)"=w504, "error in"=w507, "VISA Session In"=w508) -> ("error out"=w506:errorcluster, "Software Version"=w503:u8, "VISA Session Out"=w505:refnum<visa-resource-name>)  [unwired: 6 in]
      n283 = call "Read Controller Info.vi"("Unit ID (A)"=w504, "error in"=w506, "Software Version"=w503, "VISA Session In"=w505) -> ("error out"=w511:errorcluster, "Controller Info out"=w510:T11, "VISA Session Out"=w512:refnum<visa-resource-name>)  [unwired: 4 in, 1 out]
    }
    n284 = while {
      shift-right: [w575] -> _
      shift-left: 0.0 ("Set Start Time (s)") -> [w578]
      shift-right: [w559] -> w37
      shift-left: w18 -> [w577]
      shift-right: [w560] -> w38
      shift-left: w19 -> [w576]
      tunnel: w20 -> [w552]
      shift-right: [w563] -> _
      shift-left: w21 -> [w570]
      shift-right: [w558] -> _
      shift-left: w17 -> [w556]
      shift-right: [w554] -> _
      shift-left: w16 -> [w553]
      shift-right: [w548] -> _
      shift-left: w13 -> [w548]
      tunnel: w9 -> [w546]
      stop <- w547 stop-if-true
      # "Set minimum time\nbetween loops"
      # "Acquire data for every device ID included at the requested data rate, then display only the selected device's data"
      n285 = call "Elapsed Time"("Set Start Time (s)"=w578) -> ("Get Start Time (s)"=w575:dbl, "Elapsed Time (s)"=w572:dbl)  [unwired: 11 in, 6 out]
      n286 = Wait (ms)(milliseconds to wait="Minimum time between \nreadings [ms] (all units)") -> ()  [unwired: 1 out]
      n287 = for {
        shift-right: [w607] -> w569
        shift-left: w577 -> [w610]
        shift-right: [w608] -> w568
        shift-left: w576 -> [w609]
        tunnel: w570 -> [w604] mode=indexing
        tunnel: w552 -> [w603] mode=indexing
        tunnel: [w602] -> w567 mode=indexing
        tunnel: [w601] -> w566 mode=indexing
        tunnel: [w600] -> w565 mode=indexing
        tunnel: [w599] -> w564 mode=indexing
        tunnel: [w598] -> w563 mode=indexing
        # "Acquire data for each device"
        n288 = call "Read Measurements.vi"("error in"=w610, "Data Frame Format In"=w604, "Unit ID (A)"=w603, "VISA Session In"=w609) -> ("error out"=w607:errorcluster, "Data Frame Format Out"=w598:T10, "Data Cluster"=w601:T3, "VISA Session Out"=w608:refnum<visa-resource-name>, "Unknown Dataframe Info"=w606:bool, "Error/Overrange/Unknown String"=w600:string, "Error Present"=w605:bool, "Range Exceeded"=w599:bool)
        n289 = Or(x=w606, y=w605) -> (x .or. y?=w602:bool)
      }
      n290 = Multiply(x=1000.0 ("y"), y=w572) -> (x*y=→"Elapsed Time [ms]\n(all units)":dbl)
      n291 = Reciprocal(x=w572) -> ()  [unwired: 1 out]
      n292 = local read "Z"() -> (w542:dbl[])
      n293 = Index Array(array=w542, index=1 ("index (row)")) -> (element=w540:dbl)
      "Active Device" <- w540
      n294 = To Long Integer(number=w540) -> (32bit integer=w550:i32)
      n295 = for {
        tunnel: w569 -> [w581]
        tunnel: [w580] -> w561
        tunnel: w568 -> [w582]
        tunnel: [w579] -> w562
        tunnel: w567 -> [w587] mode=indexing
        tunnel: w550 -> [w589]
        tunnel: w566 -> [w586] mode=indexing
        tunnel: w565 -> [w585] mode=indexing
        tunnel: w564 -> [w584] mode=indexing
        i -> [w588]
        # "Iterate over all sets of data, only display the one selected"
        n296 = Equal?(x=w589, y=w588) -> (x = y?=w583:bool)
        n297 = case shown="True" w583 {
          tunnel: w587 -> [_ w597]
          tunnel: w586 -> [_ w592]
          tunnel: w585 -> [_ w596]
          tunnel: w584 -> [_ w595]
          tunnel: w582 -> [w591 w593]
          tunnel: w581 -> [w590 w594]
          tunnel: [w590 w594] -> w580
          tunnel: [w591 w593] -> w579
          frame False {
            # "Do nothing"
          }
          frame True {
            # "Display data"
            "Range Exceeded" <- w595
            "Error Present" <- w597
            "Error Text" <- w596
            "Meas. Data (for active device)" <- w592
          }
        }
      }
      n298 = Index Array(array=w548, index=w550) -> (element=w549:u8)
      n299 = local read "Z"() -> (w545:dbl[])
      n300 = Index Array(array=w552, index=w550) -> (element=w551:string)
      n301 = Index Array(array=w556, index=w550) -> (element=w555:T11)
      n302 = Index Array(array=w553, index=w550) -> (element=w539:dbl)
      n303 = Index Array(array=w545, index=0) -> (element=w543:dbl)
      n304 = call "Write SetPoint_no prev.vi"("Setpoint"=w543, "Previous Setpoint"=w539, "Unit ID (A)"=w551, "error in"=w561, "Software Version"=w549, "Controller Info out"=w555, "VISA Session In"=w562) -> ("error out"=w559:errorcluster, "Controller Info out"=w557:T11, "VISA Session Out"=w560:refnum<visa-resource-name>)  [unwired: 1 in, 1 out]
      n305 = Replace Array Subset(array=w553, new element=w543, index=w550) -> (w554:dbl[])
      n306 = Replace Array Subset(array=w556, new element=w557, index=w550) -> (w558:T12)
      n307 = call <extravilib>:"Read.vi"("channel"=w546) -> ("element"=w547:bool)  [unwired: 1 in, 1 out]
    }
    n308 = call-poly <vilib>:"Write Delimited Spreadsheet.vi"("file path (dialog if empty)"="Write File", "1D data"=string[] ["Date", "Time [hh:mm:ss]", "Device ID", "Abs_P_MFC [psi]", "T_MFC [C]", "Volume Flow [LPM]", "Mass Flow [SLPM]", "SP_MFC [LPM]", "T_SCh", "Iter_#", "V_D", "V_H", "", ""], "append to file? (new file:F)"=FALSE, "delimiter (\\t)"="," ("delimiter (\\t)")) -> ()  [unwired: 10 in, 2 out]
    n309 = VISA Close(VISA resource name=w38, error in (no error)=w37) -> (error out=w39:errorcluster)
    n310 = call <vilib>:"Simple Error Handler.vi"("error in (no error)"=w39) -> ()  [unwired: 4 in, 5 out]
    n311 = Initialize Array(0.0 ("element"), 2 ("dimension size")) -> (→"Z":dbl[])
    n312 = while "Hold Setpoints" {
      tunnel: w9 -> [w48]
      stop <- w49 stop-if-true
      n313 = call-poly <vilib>:"Read Delimited Spreadsheet.vi"("file path (dialog if empty)"="Read File", "start of read offset (chars.:0)"=0, "delimiter (\\t)"="," ("delimiter (\\t)")) -> ("all rows"=w46:dbl[][])  [unwired: 7 in, 5 out]
      "Setpoints" <- w46
      n314 = Array Size(array=w46) -> (size(s)=w51:i32[])
      n315 = call <extravilib>:"Read.vi"("channel"=w48) -> ("element"=w49:bool)  [unwired: 1 in, 1 out]
      n316 = Index Array(array=w51, index=0) -> (element=→"len_SP":i32)
    }
    n317 = node-c288(w42) -> ()  [unwired: 1 out]
  }
